vi "PrefixRemover.vi"(1 "Atto":dbl, 2 "Femto":dbl, 3 "Pico":dbl, 4 "Nano":dbl) -> (0 "No prefix":dbl)   [LabVIEW 2017]
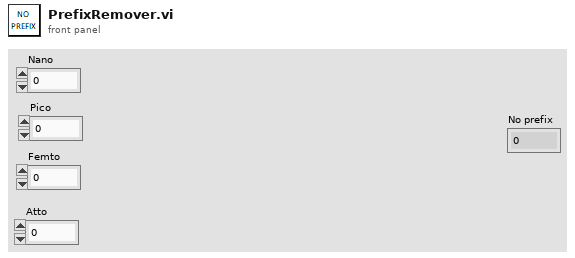
[diagram p1: front panel]
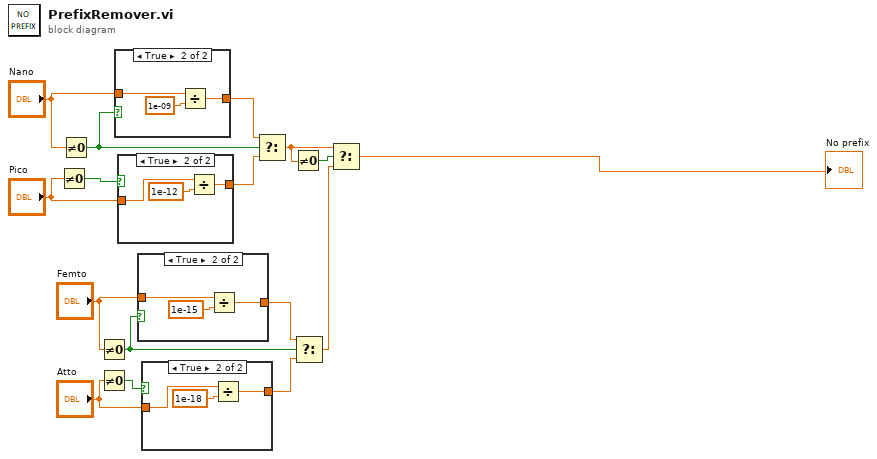
[diagram p0: block diagram]
diagram:
  n1 = Not Equal To 0?(x="Pico") -> (x != 0?=w13:bool)
  n2 = Not Equal To 0?(x="Nano") -> (x != 0?=w14:bool)
  n3 = Not Equal To 0?(x="Femto") -> (x != 0?=w7:bool)
  n4 = Not Equal To 0?(x="Atto") -> (x != 0?=w8:bool)
  n5 = case shown="True" w14 {
    tunnel: "Nano" -> [_ w18]
    tunnel: [_ w17] -> w15
    frame False {
    }
    frame True {
      n6 = Divide(x=w18, y=1e-09) -> (x/y=w17:dbl)
    }
  }
  n7 = case shown="True" w13 {
    tunnel: "Pico" -> [_ w21]
    tunnel: [_ w20] -> w11
    frame False {
    }
    frame True {
      n8 = Divide(x=w21, y=1e-12) -> (x/y=w20:dbl)
    }
  }
  n9 = case shown="True" w7 {
    tunnel: "Femto" -> [_ w24]
    tunnel: [_ w23] -> w6
    frame False {
    }
    frame True {
      n10 = Divide(x=w24, y=1e-15) -> (x/y=w23:dbl)
    }
  }
  n11 = case shown="True" w8 {
    tunnel: "Atto" -> [_ w27]
    tunnel: [_ w26] -> w5
    frame False {
    }
    frame True {
      n12 = Divide(x=w27, y=1e-18) -> (x/y=w26:dbl)
    }
  }
  n13 = Select(t=w15, s=w14, f=w11) -> (s? t:f=w3:dbl)
  n14 = Not Equal To 0?(x=w3) -> (x != 0?=w4:bool)
  n15 = Select(t=w6, s=w7, f=w5) -> (s? t:f=w2:dbl)
  n16 = Select(t=w3, s=w4, f=w2) -> (s? t:f=→"No prefix":dbl)
